vi "test.vi"() -> ()   [LabVIEW 2025, in "Power Supply.lvlib" / "PSP-603.lvclass"]
uses:
  PSP-603.lvclass
  <vilib>/Instr/_visa.llb/VISA Open Access Mode.ctl
  <vilib>/Handler Framework/CmdQueue/Enqueue Single.vi
  <vilib>/Instr/_visa.llb/VISA Configure Serial Port (Instr).vi
  PSP-603.lvclass/PSP-603.ctl
  <vilib>/Handler Framework/Handler Framework.lvlib
panel:
  out "read buffer":string
  in  "Read Status":bool
  out "resulting string":string
  in  "Set Voltage":bool
  in  "Voltage":dbl format="%05.2g"
  in  "Boolean":bool
  in  "VISA resource name":refnum<visa-resource-name>="COM13"
  out "error out":errorcluster {"code" format="%.0x"}
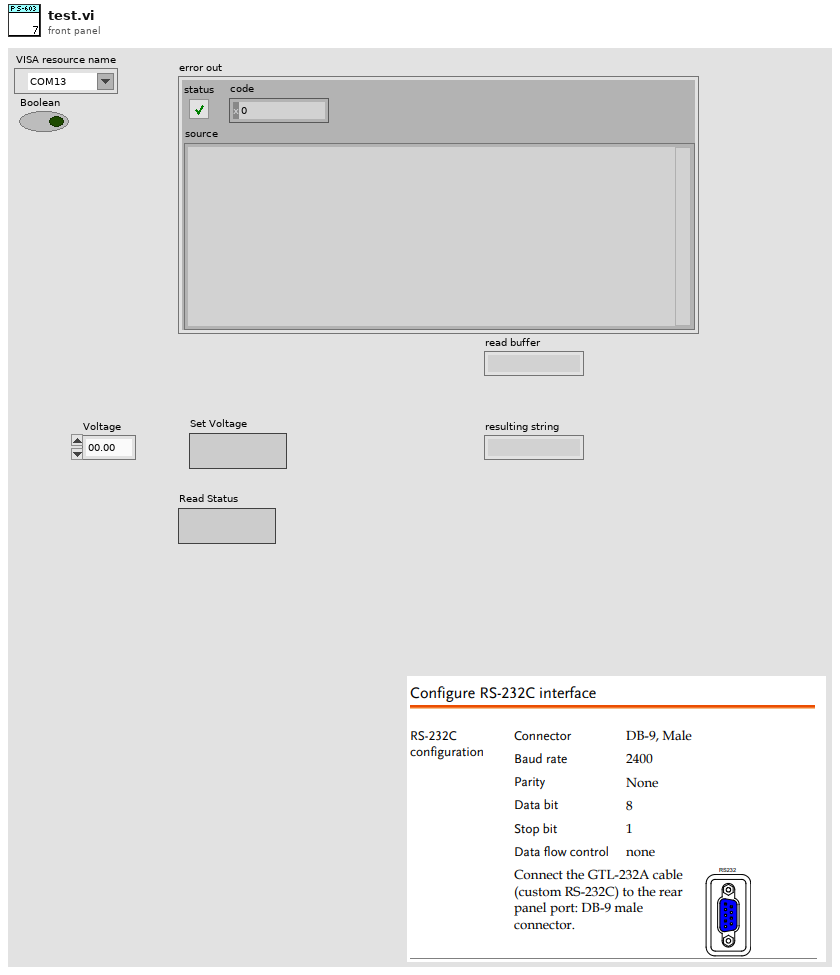
[diagram p1: front panel]
types:
  T1 = typedef "VISA Open Access Mode.ctl" = u32
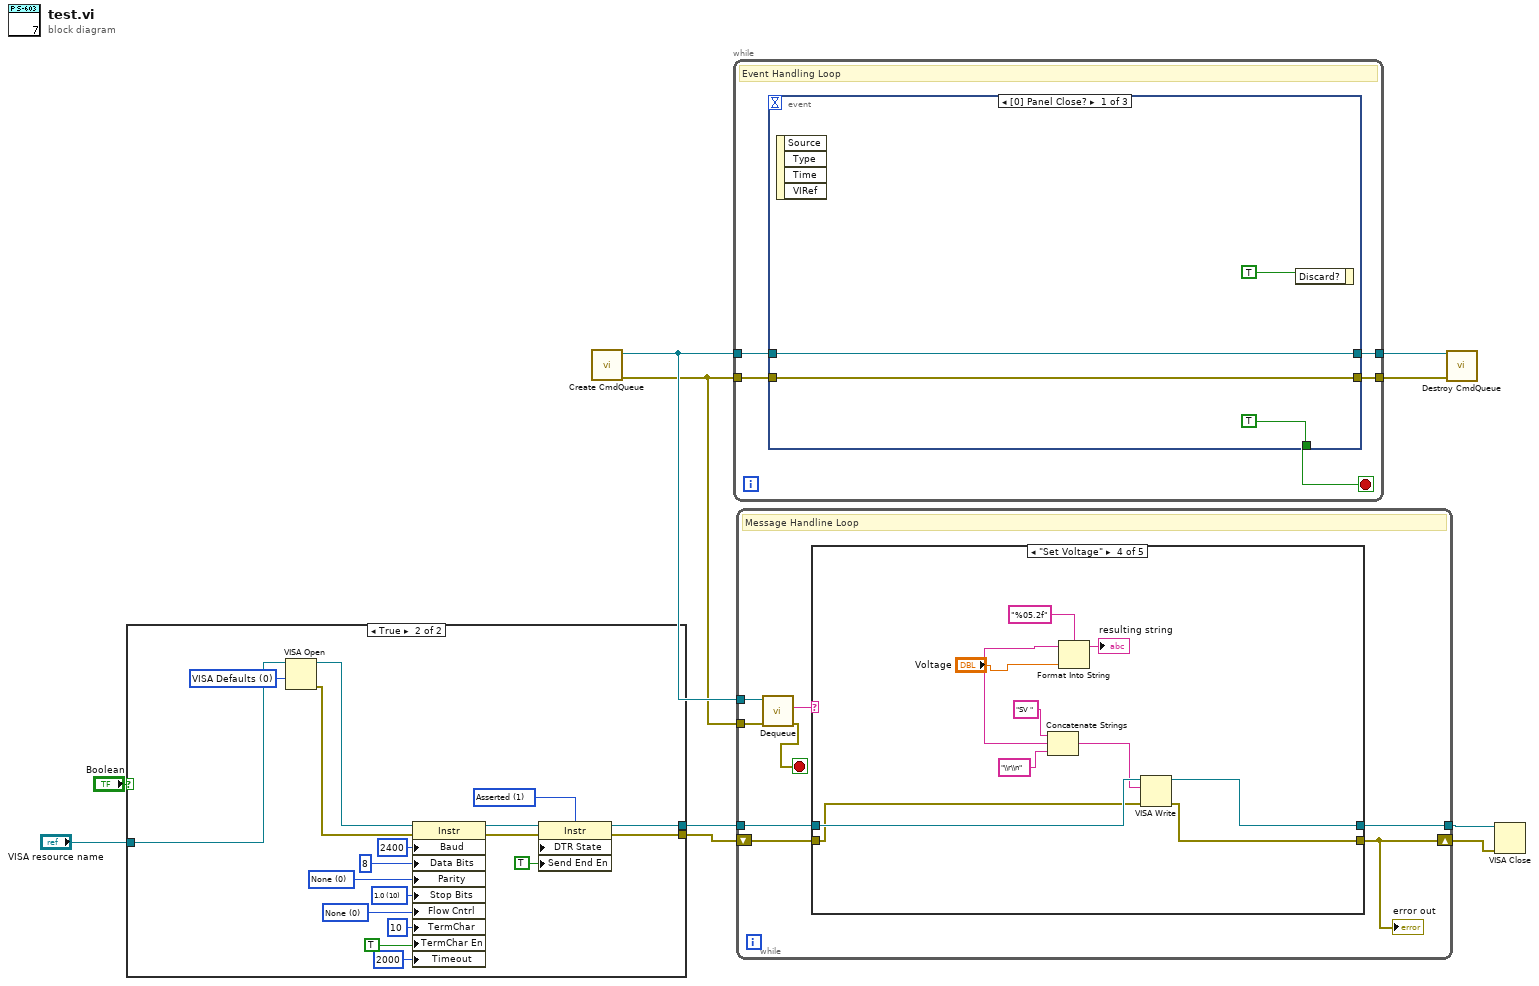
[diagram p0: block diagram]
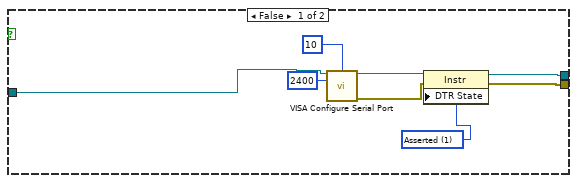
[diagram p2: hidden frame]
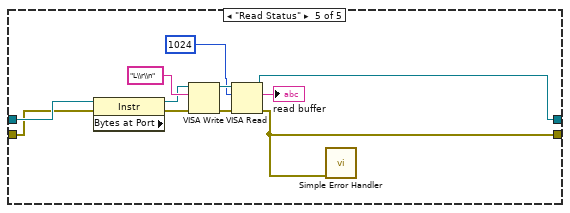
[diagram p6: hidden frame]
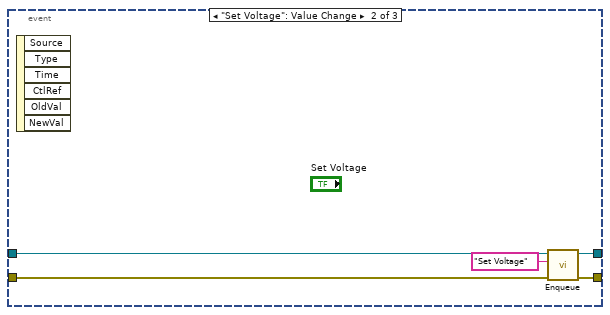
[diagram p7: hidden frame]
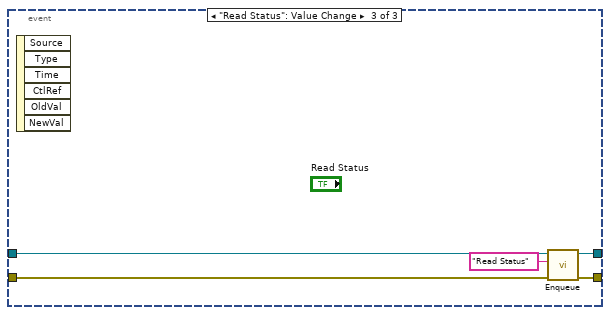
[diagram p8: hidden frame]
diagram:
  n1 = case shown="True" "Boolean" {
    tunnel: [w13 w25] -> w6
    tunnel: "VISA resource name" -> [w11 w29]
    tunnel: [w12 w24] -> w4
    frame False {
      w16 = i16 1 items=["Unknown"=-1, "Unasserted"=0, "Asserted"=1] ("Serial Settings:Modem Line Settings:Line DTR State")
      n2 = call-poly "VISA Configure Serial Port"("VISA resource name"=w11, "termination char\n(0xA = '\\n' = LF)"=u8 10 ("termination char\n(0xA = '\\n' = LF)"), "baud rate (9600)"=u32 2400) -> ("VISA resource name out"=w17:refnum<visa-resource-name>, "error out"=w18:errorcluster)  [unwired: 11 in]
      n3 = property class="Instr"(reference=w17, error in=w18, "DTR State"=w16) -> (reference out=w13:refnum<visa-resource-name>, error out=w12:errorcluster)
    }
    frame True {
      w23 = i16 1 items=["Unknown"=-1, "Unasserted"=0, "Asserted"=1] ("Serial Settings:Modem Line Settings:Line DTR State")
      w30 = u16 0 items=["None", "XON/XOFF", "RTS/CTS", "XON/XOFF & RTS/CTS", "DTR/DSR", "XON/XOFF & DTR/DSR"] ("Serial Settings:Flow Control")
      w31 = u16 10 items=["1.0"=10, "1.5"=15, "2.0"=20] ("Serial Settings:Stop Bits")
      w32 = u16 0 items=["None", "Odd", "Even", "Mark", "Space"] ("Serial Settings:Parity")
      w35 = T1 0 items=["VISA Defaults"=0, "Exclusive Lock"=1, "Load Configured Settings"=4] ("Access Mode")
      n4 = VISA Open(access mode=w35, VISA resource name=w29) -> (VISA resource name=w36:refnum<visa-resource-name>, error out=w28:errorcluster)  [unwired: 3 in]
      n5 = property class="Instr"(reference=w36, error in=w28, "Baud"=u32 2400 ("Serial Settings:Baud Rate"), "Data Bits"=u16 8 ("Serial Settings:Data Bits"), "Parity"=w32, "Stop Bits"=w31, "Flow Cntrl"=w30, "TermChar"=u8 10 ("Message Based Settings:Termination Character"), "TermChar En"=TRUE ("Message Based Settings:Termination Character Enable"), "Timeout"=u32 2000 ("General Settings:Timeout Value")) -> (reference out=w27:refnum<visa-resource-name>, error out=w26:errorcluster)
      n6 = property class="Instr"(reference=w27, error in=w26, "DTR State"=w23, "Send End En"=TRUE ("Message Based Settings:Send End Enable")) -> (reference out=w25:refnum<visa-resource-name>, error out=w24:errorcluster)
    }
  }
  n7 = call <vilib>:"Create CmdQueue.vi"() -> ("error out"=w9:errorcluster, "CmdQueue out"=w10:refnum<queue>)  [unwired: 10 in]
  n8 = while {
    tunnel: w10 -> [w40]
    tunnel: w9 -> [w39]
    tunnel: [w38] -> w8
    tunnel: [w37] -> w7
    stop <- w41 stop-if-true
    # "Event Handling Loop"
    n9 = event shown="[0] Panel Close?" {
      selector: _ -> [_ _ _]
      dyn-events: _ -> [_ _ _]
      timeout: _ -> [_ _ _]
      tunnel: [TRUE _ _] -> w41
      tunnel: w40 -> [w43 w48 w53]
      tunnel: w39 -> [w42 w47 w52]
      tunnel: [w43 w49 w54] -> w38
      tunnel: [w42 w50 w55] -> w37
      event Panel Close? {
        n10 = event-data() -> ()  [unwired: 1 in, 4 out]
        n11 = event-data("Discard?"=TRUE) -> ()  [unwired: 1 in, 1 out]
      }
      event "Set Voltage": Value Change {
        n12 = event-data() -> ()  [unwired: 1 in, 6 out]
        n13 = call-poly <vilib>:"Enqueue.vi"("error in (no error)"=w47, "Command"="Set Voltage", "CmdQueue in"=w48) -> ("error out"=w50:errorcluster, "CmdQueue out"=w49:refnum<queue>)  [unwired: 7 in]
      }
      event "Read Status": Value Change {
        n14 = event-data() -> ()  [unwired: 1 in, 6 out]
        n15 = call-poly <vilib>:"Enqueue.vi"("error in (no error)"=w52, "Command"="Read Status", "CmdQueue in"=w53) -> ("error out"=w55:errorcluster, "CmdQueue out"=w54:refnum<queue>)  [unwired: 7 in]
      }
    }
  }
  n16 = while {
    tunnel: w10 -> [w63]
    tunnel: w9 -> [w62]
    tunnel: w6 -> [w59]
    tunnel: [w58] -> w2
    shift-right: [w56] -> w1
    shift-left: w4 -> [w57]
    stop <- w61 stop-if-true
    # "Message Handline Loop"
    n17 = call <vilib>:"Dequeue.vi"("error in (no error)"=w62, "CmdQueue in"=w63) -> ("error out"=w61:errorcluster, "cmd"=w60:string)  [unwired: 5 in, 3 out]
    n18 = case shown="\"Set Voltage\"" w60 {
      tunnel: [w64 w66 w69 w76 w90] -> w58
      tunnel: w59 -> [w64 w66 w69 w77 w87]
      tunnel: w57 -> [w65 w67 w68 w75 w86]
      tunnel: [w65 w67 w68 w74 w81] -> w56
      frame Default {
      }
      frame "init" {
      }
      frame "shutdown" {
      }
      frame "Set Voltage" {
        n19 = Format Into String(format string="%05.2f", "Voltage") -> (resulting string=w72:string)  [unwired: 2 in, 1 out]
        "resulting string" <- w72
        n20 = Concatenate Strings("SV " ("string"), w72, "\\r\\n" ("string")) -> (w70:string)
        n21 = VISA Write(VISA resource name=w77, write buffer=w70, error in (no error)=w75) -> (VISA resource name out=w76:refnum<visa-resource-name>, error out=w74:errorcluster)  [unwired: 1 out]
      }
      frame "Read Status" {
        n22 = property class="Instr" props=["Bytes at Port"](reference=w87, error in=w86) -> (reference out=w83:refnum<visa-resource-name>, error out=w82:errorcluster)  [unwired: 1 out]
        n23 = VISA Write(VISA resource name=w83, write buffer="L\\r\\n", error in (no error)=w82) -> (VISA resource name out=w85:refnum<visa-resource-name>, error out=w84:errorcluster)  [unwired: 1 out]
        n24 = VISA Read(VISA resource name=w85, byte count=u32 1024, error in (no error)=w84) -> (VISA resource name out=w90:refnum<visa-resource-name>, read buffer=→"read buffer":string, error out=w81:errorcluster)  [unwired: 1 out]
        n25 = call <vilib>:"Simple Error Handler.vi"("error in (no error)"=w81) -> ()  [unwired: 4 in, 5 out]
      }
    }
    "error out" <- w56
  }
  n26 = call <vilib>:"Destroy CmdQueue.vi"("error in (no error)"=w7, "CmdQueue in"=w8) -> ()  [unwired: 9 in, 1 out]
  n27 = VISA Close(VISA resource name=w2, error in (no error)=w1) -> ()  [unwired: 1 out]
